vi "p9ctl.vi"(6 "p9 action":T1=enum."change path", 7 "ctl path":path, 10 "message":string="message", 11 "sweep folder path":path) -> (0 "ctl":string="ctl", 1 "news?":bool=TRUE, 3 "9ctl OK":bool)   [LabVIEW 2015]
uses:
  p9action control.ctl
  <vilib>/Utility/error.llb/whitespace.ctl
  ctl -- name dispatcher -- action.ctl
  file -- read-write control.ctl
  file -- 9w path.vi
  <vilib>/Utility/file.llb/Write To Spreadsheet File (string).vi
panel:
  out "path out":path
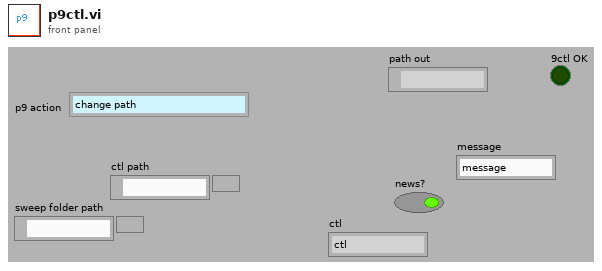
[diagram p1: front panel]
types:
  T1 = typedef "p9action control.ctl" = enum16{"init", "check", "reset", "log", "message", "change path"}
  T2 = typedef "whitespace.ctl" = u16
  T3 = typedef "ctl -- name dispatcher -- action.ctl" = enum16{"peak frequency", "peak frequency DUMP", "peak gamma DUMP", "peak gamma", "peak frequency TEST", "peak gamma TEST", "ultrasonic power", "time in gamma", "set temperature ", "set temperature timer", "peak default gamma", "last scan file", "peak freq gamma TEST", "peak NAMES", "errors", "P_I_D", "P", "I", "D", "power vs time", "power vs time TIMER", "void", "power log", "set temperature - SINE", "itc ltc log", "peak - time in gamma"}
  T4 = typedef "file -- read-write control.ctl" = enum16{"read", "write all", "append one line"}
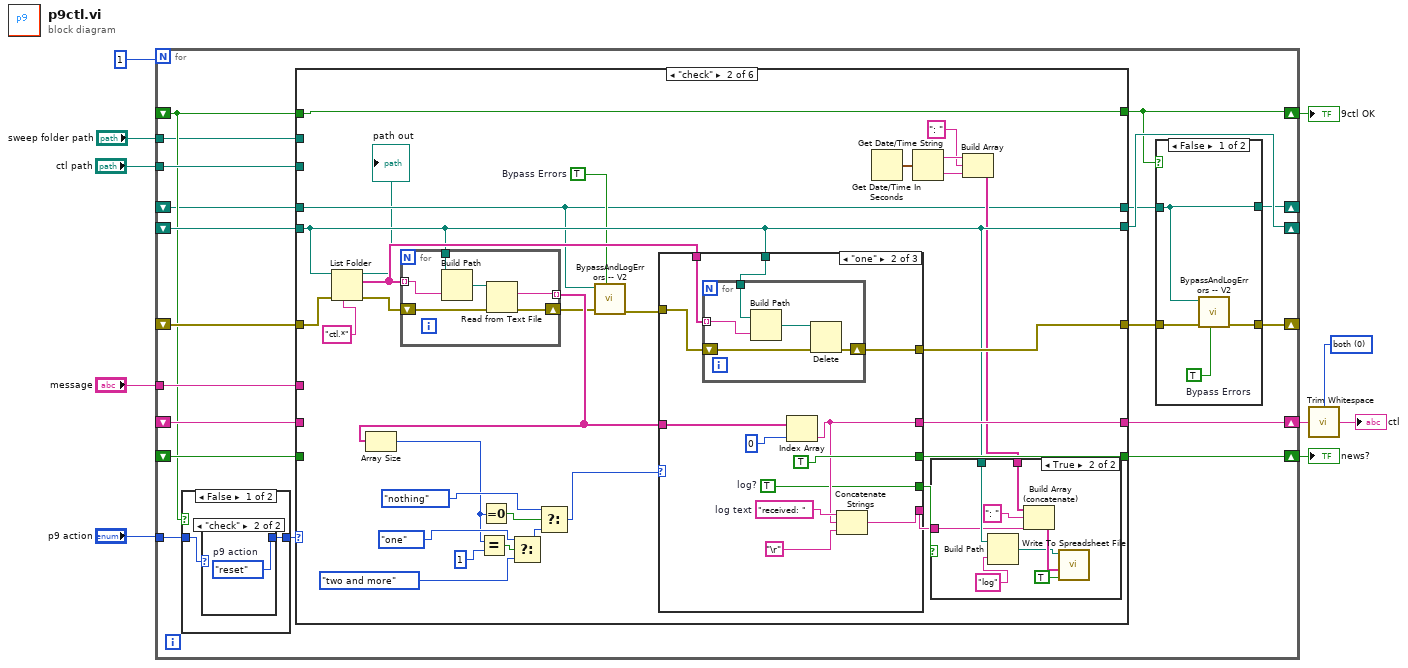
[diagram p0: block diagram]
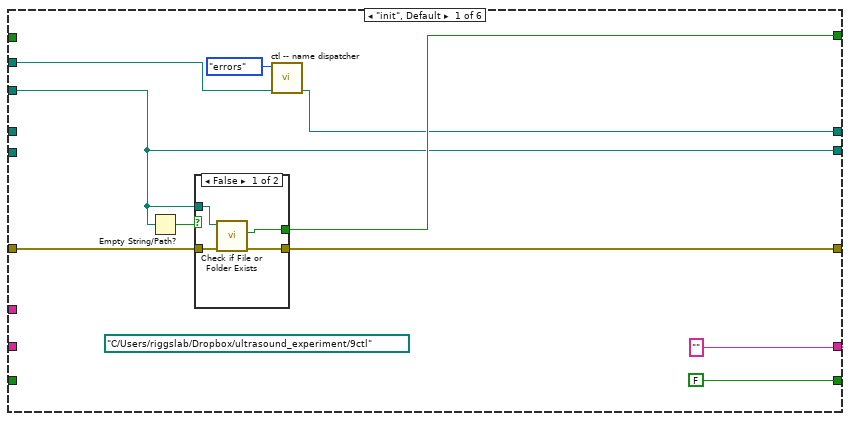
[diagram p5: hidden frame]
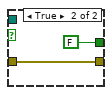
[diagram p6: hidden frame]
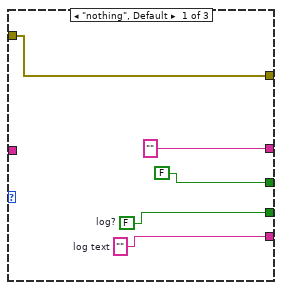
[diagram p8: hidden frame]
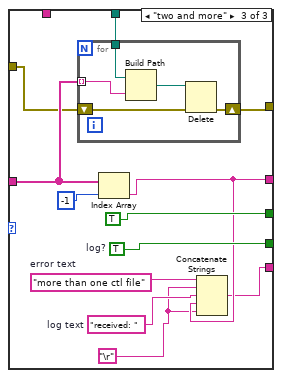
[diagram p9: hidden frame]
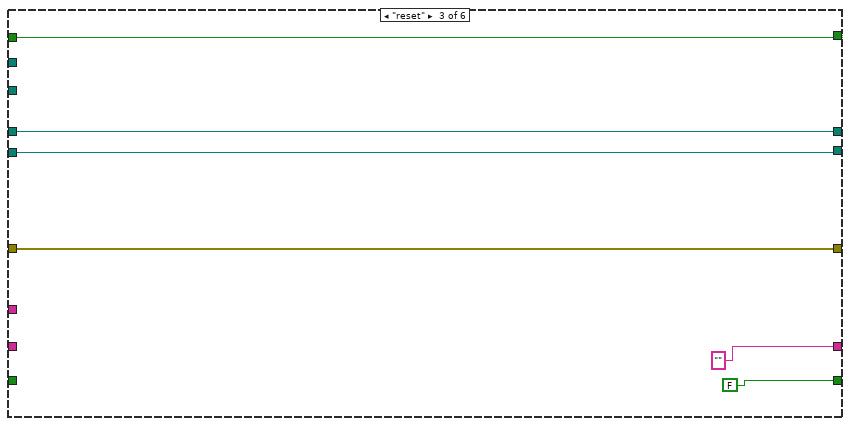
[diagram p10: hidden frame]
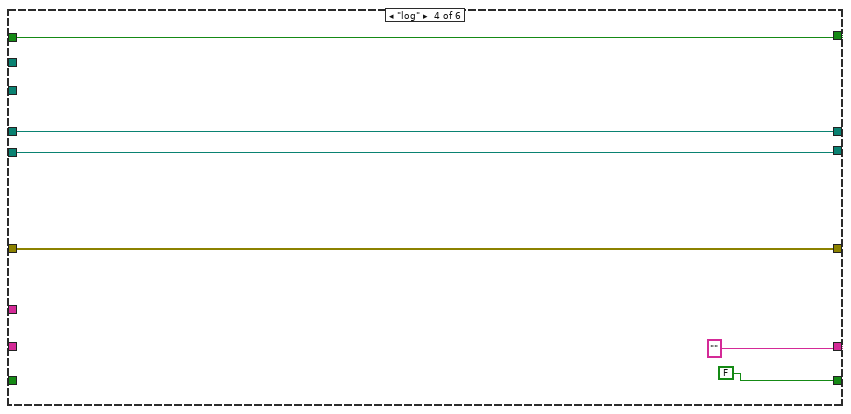
[diagram p11: hidden frame]
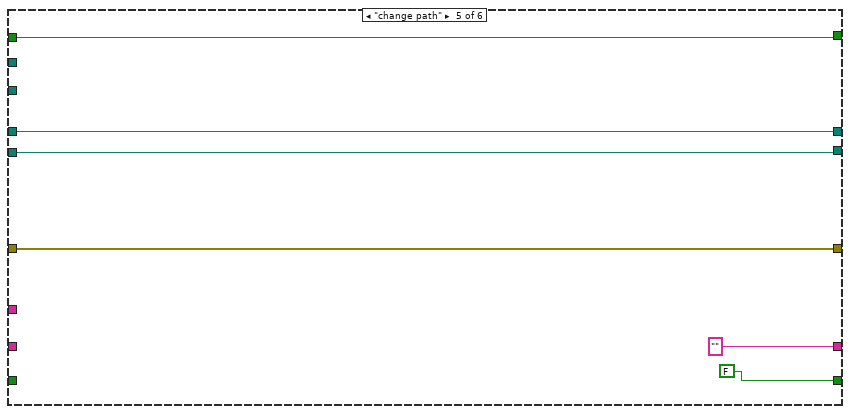
[diagram p12: hidden frame]
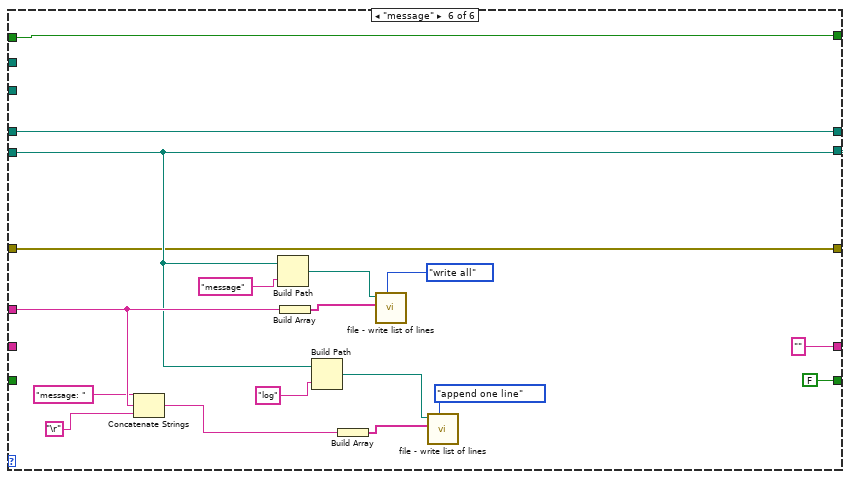
[diagram p13: hidden frame]
diagram:
  w4 = T2 0 items=["both", "start of string", "end of string"] ("location (both)")
  n1 = for {
    N: 1 -> [_]
    tunnel: "p9 action" -> [w15]
    tunnel: "ctl path" -> [w29]
    shift-right: [w19] -> _
    shift-left: _ -> [w28]
    shift-right: [w27] -> w9
    shift-left: _ -> [w23]
    shift-right: [w26] -> w6
    shift-left: _ -> [w24]
    tunnel: "message" -> [w25]
    shift-right: [w21] -> _
    shift-left: _ -> [w20]
    shift-right: [w18] -> w3
    shift-left: _ -> [w17]
    tunnel: "sweep folder path" -> [w14]
    shift-right: [w12] -> _
    shift-left: _ -> [w11]
    n2 = case shown="False" w17 {
      tunnel: [w31 w34] -> w16
      tunnel: w15 -> [w30 w34]
      frame False {
        n3 = case shown="\"check\"" w30 {
          selector: w30 -> [w32 _]
          tunnel: [w32 w33] -> w31
          frame "init", Default {
          }
          frame "check" {
            w33 = p9action_control."reset"  # p9 action
          }
        }
      }
      frame True {
      }
    }
    n4 = case shown="\"check\"" w16 {
      tunnel: [w44 w68 w146 w150 w158 w170] -> w19
      tunnel: w29 -> [w44 _ _ _ _ _]
      tunnel: w28 -> [_ w68 w146 w150 w158 w170]
      tunnel: [FALSE w78 FALSE FALSE FALSE FALSE] -> w27
      tunnel: ["" w77 "" "" "" ""] -> w26
      tunnel: w25 -> [_ _ _ _ _ w174]
      tunnel: w24 -> [_ _ _ _ _ _]
      tunnel: w23 -> [_ _ _ _ _ _]
      tunnel: [w46 w71 w143 w149 w155 w167] -> w22
      tunnel: w20 -> [w48 w70 w143 w149 w155 w167]
      tunnel: [w45 w59 w142 w148 w154 w166] -> w18
      tunnel: w17 -> [_ w59 w142 w148 w154 w166]
      tunnel: w14 -> [w43 _ _ _ _ _]
      tunnel: [w41 w58 w141 w147 w153 w165] -> w13
      tunnel: w11 -> [_ w58 w141 w147 w153 w165]
      frame "init", Default {
        (unwired) path "C:/Users/riggslab/Dropbox/ultrasound_experiment/9ctl"
        n5 = Empty String/Path?(string/path=w44) -> (empty?=w47:bool)
        n6 = case shown="False" w47 {
          tunnel: w48 -> [w54 w55]
          tunnel: [w53 w55] -> w46
          tunnel: w44 -> [w52 _]
          tunnel: [w51 FALSE] -> w45
          frame False {
            n7 = call <vilib>:"Check if File or Folder Exists.vi"("error in (no error)"=w54, "path"=w52) -> ("error out"=w53:errorcluster, "file or folder exists?"=w51:bool)  [unwired: 7 in, 1 out]
          }
          frame True {
          }
        }
        n8 = call "ctl -- name dispatcher.vi"("sweep folder path"=w43, "ctl name dispatch"=ctl_--_name_dispatcher_--_action."errors" ("ctl kind")) -> ("file path"=w41:path)  [unwired: 7 in, 2 out]
      }
      frame "check" {
        w67 = TRUE  # Bypass Errors
        n9 = List Folder(path=w68, pattern="ctl.*", error in=w70) -> (path out=→"path out":path, filenames=w72:string[], error out=w69:errorcluster)  [unwired: 1 in, 1 out]
        n10 = for {
          tunnel: w72 -> [w140] mode=indexing
          tunnel: w68 -> [w139]
          tunnel: [w137] -> w74 mode=indexing
          shift-right: [w136] -> w66
          shift-left: w69 -> [w135]
          n11 = Build Path(base path=w139, name or relative path=w140) -> (appended path=w138:path)
          n12 = Read from Text File(file (use dialog)=w138, error in=w135) -> (text=w137:string, error out=w136:errorcluster)  [unwired: 2 in, 2 out]
        }
        n13 = Array Size(array=w74) -> (size(s)=w73:i32)
        n14 = Equal?(x=w73, y=1) -> (x = y?=w83:bool)
        n15 = Equal To 0?(x=w73) -> (x = 0?=w85:bool)
        n16 = Select(t=enum16{"nothing", "one", "two and more"}."one" ("action"), s=w83, f=enum16{"nothing", "one", "two and more"}."two and more" ("action")) -> (s? t:f=w80:enum16{"nothing", "one", "two and more"})
        n17 = Select(t=enum16{"nothing", "one", "two and more"}."nothing" ("action"), s=w85, f=w80) -> (s? t:f=w79:enum16{"nothing", "one", "two and more"})
        n18 = call "BypassAndLogErrors -- V2.vi"("Bypass Errors"=w67, "error in (no error)"=w66, "Log File Path"=w58) -> ("error out"=w65:errorcluster)  [unwired: 8 in]
        n19 = case shown="\"one\"" w79 {
          tunnel: [FALSE TRUE TRUE] -> w78
          tunnel: ["" w107 w123] -> w77
          tunnel: w74 -> [_ w110 w127]
          tunnel: w68 -> [_ w109 w126]
          tunnel: [w98 w105 w125] -> w76
          tunnel: [w97 w104 w120] -> w75
          tunnel: w72 -> [_ w103 _]
          tunnel: w65 -> [w96 w102 w118]
          tunnel: [w96 w101 w119] -> w71
          frame "nothing", Default {
            w97 = ""  # log text
            w98 = FALSE  # log?
          }
          frame "one" {
            w108 = "received: "  # log text
            w105 = TRUE  # log?
            n20 = for {
              tunnel: w103 -> [w117] mode=indexing
              tunnel: w109 -> [w116]
              shift-right: [w113] -> w101
              shift-left: w102 -> [w114]
              n21 = Build Path(base path=w116, name or relative path=w117) -> (appended path=w115:path)
              n22 = Delete(path (use dialog)=w115, error in=w114) -> (error out=w113:errorcluster)  [unwired: 3 in, 2 out]
            }
            n23 = Index Array(array=w110, index=0) -> (element=w107:string)
            n24 = Concatenate Strings(w108, w107, "\r") -> (w104:string)
          }
          frame "two and more" {
            w121 = "\r"
            w124 = "received: "  # log text
            w122 = "more than one ctl file"  # error text
            w125 = TRUE  # log?
            n25 = for {
              tunnel: w127 -> [w134] mode=indexing
              tunnel: w126 -> [w133]
              shift-right: [w131] -> w119
              shift-left: w118 -> [w130]
              n26 = Build Path(base path=w133, name or relative path=w134) -> (appended path=w132:path)
              n27 = Delete(path (use dialog)=w132, error in=w130) -> (error out=w131:errorcluster)  [unwired: 3 in, 2 out]
            }
            n28 = Index Array(array=w127, index=-1) -> (element=w123:string)
            n29 = Concatenate Strings(w122, w121, w124, w123, w121) -> (w120:string)
          }
        }
        n30 = Get Date/Time In Seconds() -> (seconds since 1Jan1904=w64:timestamp)
        n31 = Get Date/Time String(seconds (now)=w64) -> (date string=w63:string, time string=w62:string)  [unwired: 2 in]
        n32 = Build Array(w63, ": ", w62) -> (w60:string[])
        n33 = case shown="True" w76 {
          tunnel: w68 -> [_ w95]
          tunnel: w75 -> [_ w93]
          tunnel: w60 -> [_ w88]
          frame False {
          }
          frame True {
            n34 = Build Path(base path=w95, name or relative path="log") -> (appended path=w91:path)
            n35 = Build Array (concatenate)(w88, ": ", w93) -> (w92:string[])
            n36 = call-poly <vilib>:"Write To Spreadsheet File.vi"("append to file? (new file:F)"=TRUE, "1D data"=w92, "file path (dialog if empty)"=w91) -> ()  [unwired: 5 in, 1 out]
          }
        }
      }
      frame "reset" {
      }
      frame "log" {
      }
      frame "change path" {
      }
      frame "message" {
        n37 = Concatenate Strings("message: ", w174, "\r") -> (w171:string)
        n38 = Build Path(base path=w170, name or relative path="message") -> (appended path=w159:path)
        n39 = Build Array(w174) -> (w160:string[])
        n40 = Build Path(base path=w170, name or relative path="log") -> (appended path=w163:path)
        n41 = Build Array(w171) -> (w162:string[])
        n42 = call "file - write list of lines.vi"("read/write control"=file_--_read-write_control."write all", "list of lines IN"=w160, "file path"=w159) -> ()  [unwired: 7 in, 2 out]
        n43 = call "file - write list of lines.vi"("read/write control"=file_--_read-write_control."append one line", "list of lines IN"=w162, "file path"=w163) -> ()  [unwired: 7 in, 2 out]
      }
    }
    n44 = case shown="False" w18 {
      tunnel: w22 -> [w37 w40]
      tunnel: [w36 w40] -> w21
      tunnel: [w35 w39] -> w12
      tunnel: w13 -> [w35 w39]
      frame False {
        w38 = TRUE  # Bypass Errors
        n45 = call "BypassAndLogErrors -- V2.vi"("Bypass Errors"=w38, "error in (no error)"=w37, "Log File Path"=w35) -> ("error out"=w36:errorcluster)  [unwired: 8 in]
      }
      frame True {
      }
    }
  }
  "news?" <- w9
  "9ctl OK" <- w3
  n46 = call <vilib>:"Trim Whitespace.vi"("string"=w6, "location (both)"=w4) -> ("trimmed string"=→"ctl":string)
